vi "Measure.vi"(8 "error in (no error)":errorcluster, 10 "Measure Type":i32(ring) items=["Current", "High Current", "Low Current", "Max Current", "Min Current", "Power", "Voltage", "High Voltage", "Low Voltage", "Max Voltage", "Min Voltage", "A Hour", "W Hour", "Local Voltage", "Remote Voltage"], 11 "VISA resource name":refnum<visa-resource-name>) -> (0 "error out":errorcluster, 2 "Value":dbl, 3 "VISA resource name out":refnum<visa-resource-name>)   [LabVIEW 2015, in "IT6000C.lvlib"]
doc: "The MEASure subsystem command measures the output voltage or current.These commands will trigger the acquisition of additional data before the readings are returned.Perform the measurement by digitizing the instantaneous output voltage or current at the specified measurement time, storing the result in the buffer and calculating the value of the specified measurement type.\n\n<b>Measure Type</b>\n0:Current\n1:High Current\n2:Low Current\n3:Max Current\n4:Min Current\n5:Power\n6:Voltage\n7:High Voltage\n8:Low Voltage\n9:Max Voltage\n10:Min Voltage\n11:A Hour\n12:W Hour\n13:Local Voltage\n14:Remote Voltage"
uses:
  <instrlib>/IT6000C/IT6000C.lvlib
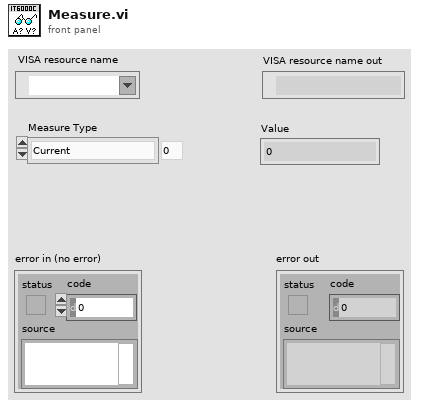
[diagram p1: front panel]
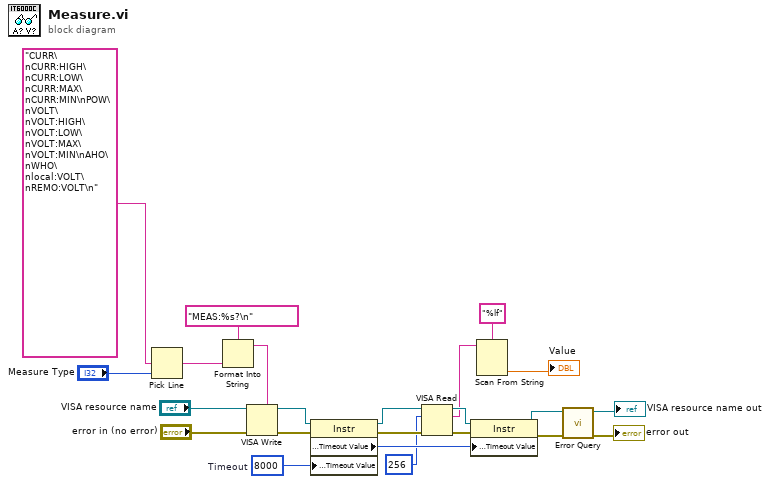
[diagram p0: block diagram]
diagram:
  w21 = u32 8000  # Timeout
  n1 = Pick Line(multi-line string="CURR\nCURR:HIGH\nCURR:LOW\nCURR:MAX\nCURR:MIN\nPOW\nVOLT\nVOLT:HIGH\nVOLT:LOW\nVOLT:MAX\nVOLT:MIN\nAHO\nWHO\nlocal:VOLT\nREMO:VOLT\n", line index="Measure Type") -> (output string=w8:string)  [unwired: 1 in]
  n2 = Format Into String(format string="MEAS:%s?\n", w8) -> (resulting string=w11:string)  [unwired: 2 in, 1 out]
  n3 = VISA Write(VISA resource name="VISA resource name", write buffer=w11, error in (no error)="error in (no error)") -> (VISA resource name out=w23:refnum<visa-resource-name>, error out=w22:errorcluster)  [unwired: 1 out]
  n4 = property class="Instr"(reference=w23, error in=w22, "General Settings:Timeout Value"=w21) -> (reference out=w16:refnum<visa-resource-name>, error out=w17:errorcluster, "General Settings:Timeout Value"=w18:u32)
  n5 = VISA Read(VISA resource name=w16, byte count=256, error in (no error)=w17) -> (VISA resource name out=w20:refnum<visa-resource-name>, read buffer=w13:string, error out=w19:errorcluster)  [unwired: 1 out]
  n6 = property class="Instr"(reference=w20, error in=w19, "General Settings:Timeout Value"=w18) -> (reference out=w1:refnum<visa-resource-name>, error out=w2:errorcluster)
  n7 = Scan From String(format string="%lf", input string=w13) -> (output 1=→"Value":dbl)  [unwired: 3 in, 3 out]
  n8 = call <instrlib>:"Error Query.vi"("error in (no error)"=w2, "VISA resource name"=w1) -> ("error out"=→"error out":errorcluster, "VISA resource name out"=→"VISA resource name out":refnum<visa-resource-name>)  [unwired: 6 in, 2 out]
